vi "Show the data.vi"(8 "error in (no error)":errorcluster, 10 "Table Name":string, 11 "Import Export in":refnum<class "Export.lvclass">) -> (0 "error out":errorcluster, 3 "Import Export out":refnum<class "Export.lvclass">)   [LabVIEW 2023, in "Data Analysis.lvlib" / "Export.lvlib" / "Export.lvclass"]
uses:
  Export.lvclass
  Export.lvclass/Export.ctl
  HardwareAbstractionLayer_LVOOP/Database/Database.lvclass
  Data Analysis.lvlib
  <vilib>/Utility/miscctls.llb/LVRowAndColumnUnsignedTypeDef.ctl
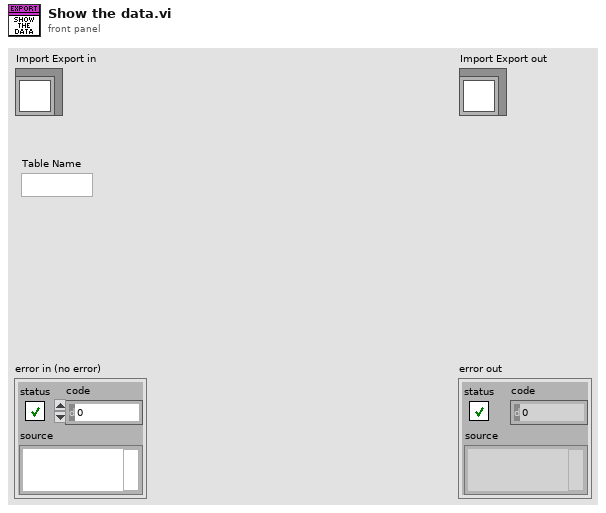
[diagram p1: front panel]
types:
  T1 = typedef "LVRowAndColumnUnsignedTypeDef.ctl" = cluster{"Row":u32, "Column":u32}
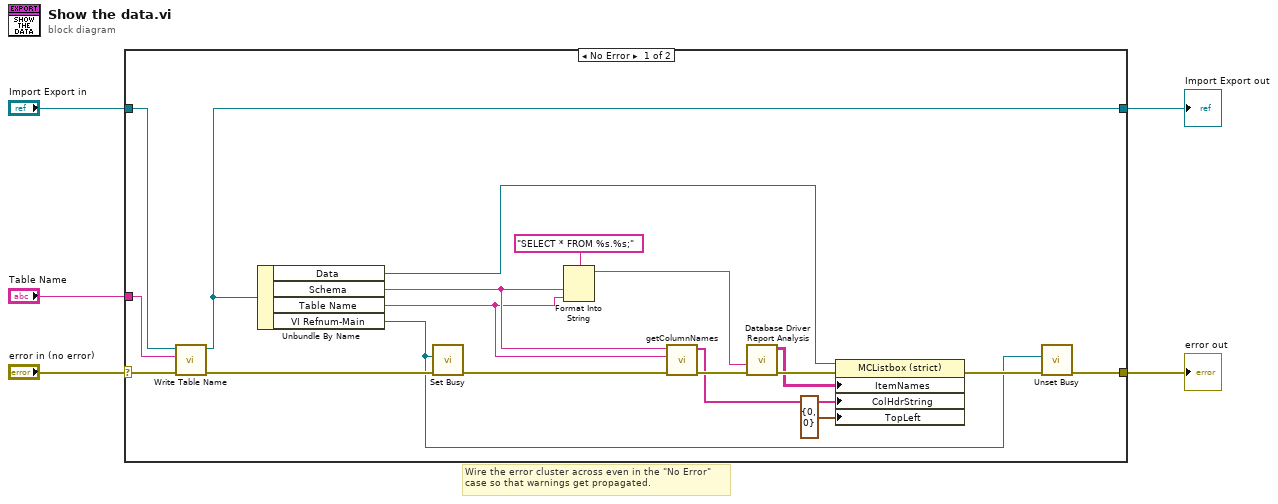
[diagram p0: block diagram]
diagram:
  # "Wire the error cluster across even in the \"No Error\"\ncase so that warnings get propagated."
  n1 = case shown="No Error" "error in (no error)" {
    selector: "error in (no error)" -> [w15 w26]
    tunnel: [w8 w26] -> w4
    tunnel: [w10 w25] -> w2
    tunnel: "Import Export in" -> [w14 w25]
    tunnel: "Table Name" -> [w13 _]
    frame No Error {
      n2 = call "Write Table Name.vi"("error in (no error)"=w15, "Table Name"=w13, "Import Export in"=w14) -> ("error out"=w12:errorcluster, "Import Export out"=w10:refnum<class "Export.lvclass">)  [unwired: 7 in]
      n3 = Unbundle By Name(w10) -> ("Data"=w18:refnum<vi>, "Schema"=w21:string, "Table Name"=w20:string, "VI Refnum-Main"=w7:refnum<vi>)
      n4 = call <vilib>:"Set Busy.vi"("error in (no error)"=w12, "VI reference (current VI)"=w7) -> ("error out"=w11:errorcluster)  [unwired: 8 in, 1 out]
      n5 = Format Into String(format string="SELECT * FROM %s.%s;", w21, w20) -> (resulting string=w23:string)  [unwired: 2 in, 1 out]
      n6 = call "getColumnNames.vi"("error in (no error)"=w11, "tableName"=w20, "schema"=w21) -> ("error out"=w22:errorcluster, "columnNames"=w16:string[])  [unwired: 6 in, 1 out]
      n7 = call "Database Driver Report Analysis.vi"("error in"=w22, "SQL query"=w23) -> ("error out"=w19:errorcluster, "data"=w17:string[][])  [unwired: 6 in, 2 out]
      n8 = property class="MCListbox (strict)"(reference=w18, error in=w19, "ItemNames"=w17, "ColHdrString"=w16, "TopLeft"=T1 {"Row"=0, "Column"=0} ("Top Left Visible Cell")) -> (error out=w9:errorcluster)  [unwired: 1 out]
      n9 = call <vilib>:"Unset Busy.vi"("error in (no error)"=w9, "VI reference (current VI)"=w7) -> ("error out"=w8:errorcluster)  [unwired: 9 in]
    }
    frame Error {
    }
  }
  "error out" <- w4
  "Import Export out" <- w2
